vi "Rectangle2006.vi"   [LabVIEW 2013]
uses:
  <vilib>/Heliosphere Research LLC/Advanced Plotting Toolkit/api_core/NewPlotProperties.ctl
  <vilib>/Heliosphere Research LLC/Advanced Plotting Toolkit/typedefs/PlotColor.ctl
  ModeType.ctl
  <vilib>/Heliosphere Research LLC/Advanced Plotting Toolkit/Advanced Plotting Toolkit.lvlib
types:
  T1 = typedef "ModeType.ctl" = enum16{"Normal", "Expected Failure", "Skipped", "Broken"}
  T2 = typedef "Advanced Plotting Toolkit.lvlib/NewPlotProperties.ctl" = cluster{"Background Color":T3, "Axis Background":T3, "Left Margin":dbl, "Right Margin":dbl, "Bottom Margin":dbl, "Top Margin":dbl, "Aspect Ratio":dbl}
  T3 = typedef "Advanced Plotting Toolkit.lvlib/PlotColor.ctl" = u32
  T4 = typedef "Advanced Plotting Toolkit.lvlib/PlotID.ctl" = i32
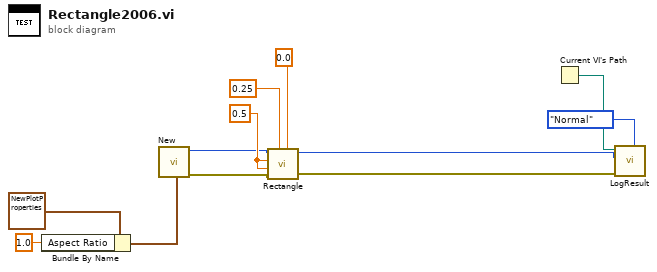
[diagram p0: block diagram]
diagram:
  w11 = 0.5 ("X Position")
  n1 = Bundle By Name(cluster=T2 {"Background Color"=2147483647, "Axis Background"=2147483647, "Left Margin"=nan, "Right Margin"=nan, "Bottom Margin"=nan, "Top Margin"=nan, "Aspect Ratio"=nan} ("New Plot Properties"), "Aspect Ratio"=1.0) -> (w5:T2)
  n2 = call <vilib>:"New.vi"("Properties"=w5) -> ("error out"=w9:errorcluster, "Plot ID"=w10:T4)  [unwired: 9 in]
  n3 = call <vilib>:"Rectangle.vi"("Height"=0.0, "Width"=0.25 ("Radius"), "error in (no error)"=w9, "Y Position"=w11, "X Position"=w11, "Plot ID"=w10) -> ("error out"=w7:errorcluster, "Plot ID Out"=w8:T4)  [unwired: 4 in]
  n4 = Current VI's Path() -> (path=w12:path)
  n5 = call "LogResult.vi"("Mode"=ModeType."Normal", "Test Result"=w7, "Test Artifact"=w8, "VI Path"=w12) -> ()  [unwired: 8 in]
